vi "LineByLine.vi"(9 "Processor":enum16{"SPIKE", "Pi"}(ring), 11 "Python Code":string) -> (3 "result string":string)   [LabVIEW 2022 SP3]
uses:
  <vilib>/Utility/error.llb/Trim Whitespace One-Sided.vi
panel:
  out "spaces at end":bool
  out "Array":cluster{"cmd":string, "indent":i32}[](array[cluster])
  out "Lines":string[](array[string])
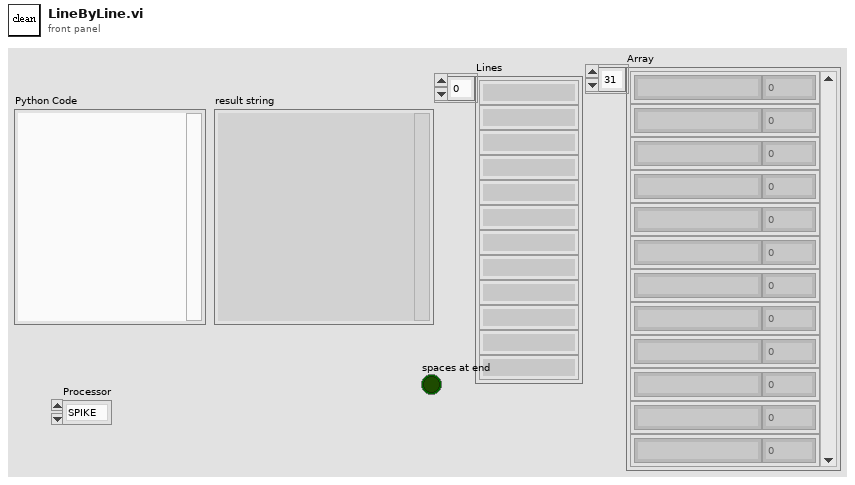
[diagram p1: front panel]
types:
  T1 = cluster{"String out":string, "number of replacements":i32}
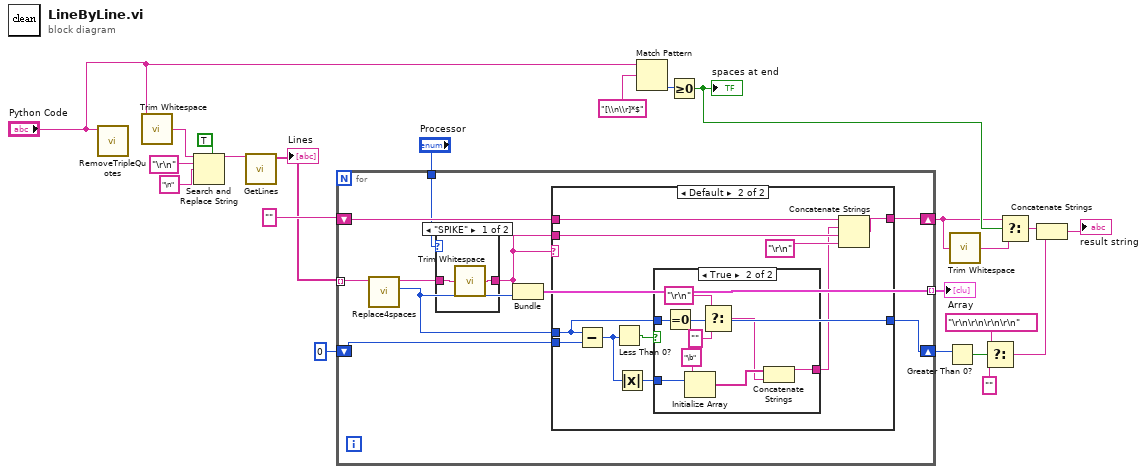
[diagram p0: block diagram]
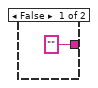
[diagram p4: hidden frame]
diagram:
  n1 = call "RemoveTripleQuotes.vi"("Python Code in"="Python Code") -> ()  [unwired: 10 in, 1 out]
  n2 = call <vilib>:"Trim Whitespace.vi"("string"="Python Code") -> ("trimmed string"=w16:string)  [unwired: 1 in]
  n3 = Search and Replace String(replace all?=TRUE ("replace all? (F)"), input string=w16, search string="\r\n" ("search"), replace string="\n" ("replace")) -> (result string=w3:string)  [unwired: 4 in, 3 out]
  n4 = call "GetLines.vi"("String"=w3) -> ("Array"=w2:string[])  [unwired: 10 in]
  "Lines" <- w2
  n5 = for {
    tunnel: w2 -> [w33] mode=indexing
    shift-right: [w27] -> w15
    shift-left: 0 ("number of replacements") -> [w32]
    shift-right: [w30] -> w6
    shift-left: "" ("format string") -> [w31]
    tunnel: [w29] -> w18 mode=indexing
    tunnel: "Processor" -> [w24]
    n6 = call "Replace4spaces.vi"("String in"=w33) -> ("number of replacements"=w28:i32, "String out"=w26:string)  [unwired: 9 in]
    n7 = case shown="\"SPIKE\"" w24 {
      tunnel: w26 -> [w34 w36]
      tunnel: [w35 w36] -> w25
      frame "SPIKE" {
        n8 = call <vilib>:"Trim Whitespace.vi"("string"=w34) -> ("trimmed string"=w35:string)  [unwired: 1 in]
      }
      frame "Pi", Default {
      }
    }
    n9 = Bundle("String out"=w25, "number of replacements"=w28) -> (w29:T1)  [unwired: 1 in]
    n10 = case shown="Default" w25 {
      tunnel: w32 -> [w37 w48]
      tunnel: w31 -> [w38 w44]
      tunnel: [w38 w43] -> w30
      tunnel: w25 -> [_ w41]
      tunnel: w28 -> [_ w40]
      tunnel: [w37 w40] -> w27
      frame "" {
      }
      frame Default {
        n11 = Subtract(x=w40, y=w48) -> (x-y=w46:i32)
        n12 = Less Than 0?(x=w46) -> (x < 0?=w47:bool)
        n13 = Absolute Value(x=w46) -> (abs(x)=w45:i32)
        n14 = case shown="True" w47 {
          tunnel: w45 -> [_ w54]
          tunnel: ["" ("delimiter (Tab)") w57] -> w39
          tunnel: w40 -> [_ w55]
          frame False {
          }
          frame True {
            n15 = Equal To 0?(x=w55) -> (x = 0?=w53:bool)
            n16 = Initialize Array("\b" ("String"), w54) -> (w58:string[])
            n17 = Select(t="\r\n" ("delimiter (Tab)"), s=w53, f="" ("delimiter (Tab)")) -> (s? t:f=w50:string)
            n18 = Concatenate Strings(w58, w50) -> (w57:string)
          }
        }
        n19 = Concatenate Strings(w44, w39, w41, "\r\n" ("delimiter (Tab)")) -> (w43:string)
      }
    }
  }
  "Array" <- w18
  n20 = Match Pattern(string="Python Code", regular expression="[\\n\\r]*$") -> (offset past match=w9:i32)  [unwired: 1 in, 3 out]
  n21 = Greater Or Equal To 0?(x=w9) -> (x >= 0?=w8:bool)
  "spaces at end" <- w8
  n22 = Greater Than 0?(x=w15) -> (x > 0?=w14:bool)
  n23 = call <vilib>:"Trim Whitespace.vi"("string"=w6) -> ("trimmed string"=w5:string)  [unwired: 1 in]
  n24 = Select(t="\r\n\r\n\r\n\r\n" ("delimiter (Tab)"), s=w14, f="" ("delimiter (Tab)")) -> (s? t:f=w13:string)
  n25 = Select(t=w6, s=w8, f=w5) -> (s? t:f=w7:string)
  n26 = Concatenate Strings(w7, w13) -> (→"result string":string)
